vi "svl_Log View for Energy Level (single value).vi"(6 "include weighting if dB On FALSE":bool=TRUE, 7 "channel info":T1={"sensor sensitivity"=1000.0, "engineering units"=0, "dB reference"=0.0, "custom label"="EU", "weighting filter"=0, "pregain"=0.0} {"pregain" format="%.2f"; "weighting filter" items=["Linear", "A-weighting", "B-weighting", "C-weighting", "ITU-R 468-4", "Dolby", "CCITT", "C-message", "Wb", "Wc", "Wd", "We", "Wf", "Wh", "Wj", "Wk", "Wm", "AES17 20 kHz lowpass", "AES17 40 kHz lowpass", "AES17 20 kHz highpass", "AES17 40 kHz highpass"]; "dB reference" format="%^.1e"; "engineering units" items=["custom..."=0, "V"=1, "A"=21, "C"=30, "pC"=31, "s"=32, "-"=29, "Pa"=2, "N"=20, "g"=3, "m/s^2"=4, "m/s"=5, "m"=6, "mm/s"=12, "mm"=13, "micron/s"=14, "micron"=15, "in/s^2"=7, "in/s"=8, "in"=9, "mil/s"=10, "mil"=11, "rad/s^2"=16, "rad/s"=17, "rad"=18, "deg/s^2"=26, "deg/s"=27, "deg"=28, "RPM"=22, "cycle/s^2"=23, "Hz"=24, "cycle"=25, "strain"=19]; "sensor sensitivity" format="%#_5f"}, 8 "error in (no error)":errorcluster, 9 "view mode":enum16{"Power", "Amplitude"}(ring), 10 "dB On (T)":bool=TRUE, 11 "energy level [EU^2 rms]":dbl format="%.2f") -> (0 "error out":errorcluster, 2 "unit label":string, 3 "energy level [EU^2 rms]":dbl format="%.2f")   [LabVIEW 2017]
uses:
  <vilib>/addons/_NISVFA/_Shared subVIs/Controls/svc_Channel Info.ctl
  <vilib>/addons/_NISVFA/_Shared subVIs/Controls/svc_Engineering Units Text Ring.ctl
  <vilib>/addons/_NISVFA/_Shared subVIs/Controls/svc_Weighting Filter Text Ring.ctl
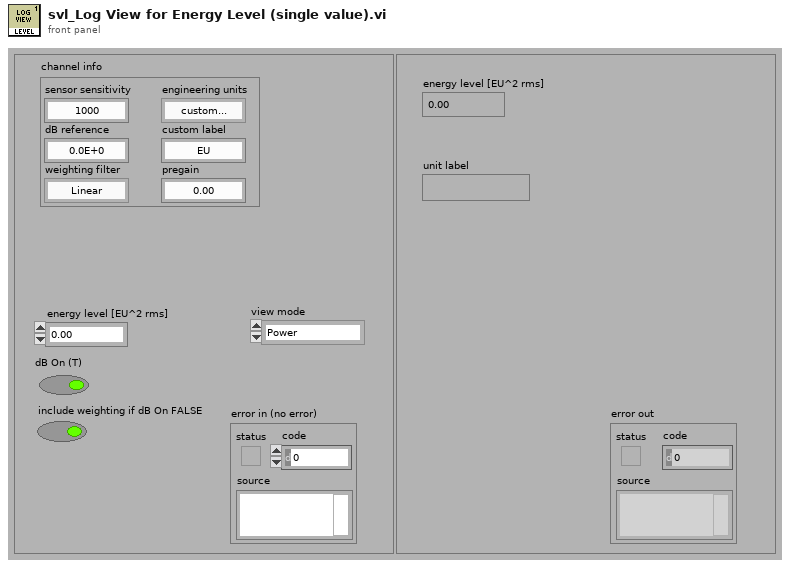
[diagram p1: front panel]
types:
  T1 = typedef "svc_Channel Info.ctl" = cluster{"sensor sensitivity":dbl, "engineering units":T2, "dB reference":dbl, "custom label":string, "weighting filter":T3, "pregain":dbl}
  T2 = typedef "svc_Engineering Units Text Ring.ctl" = u16
  T3 = typedef "svc_Weighting Filter Text Ring.ctl" = u16
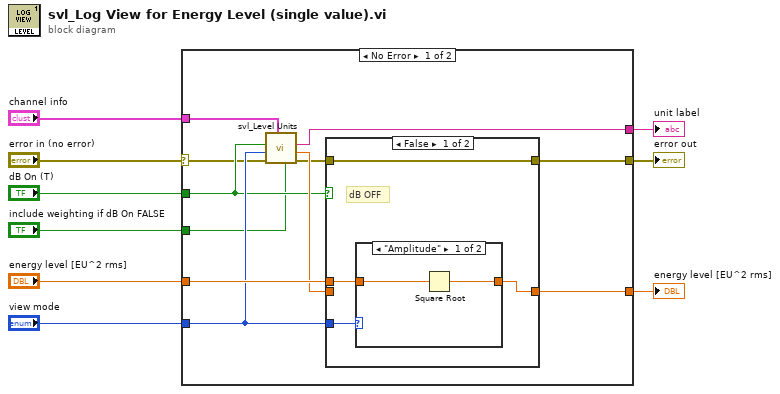
[diagram p0: block diagram]
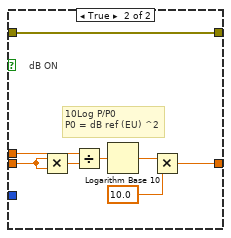
[diagram p3: hidden frame]
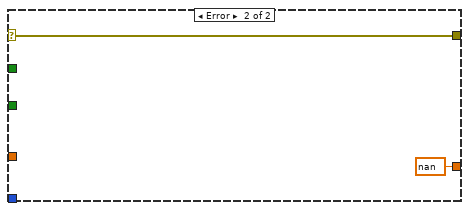
[diagram p4: hidden frame]
diagram:
  n1 = case shown="No Error" "error in (no error)" {
    selector: "error in (no error)" -> [w10 w37]
    tunnel: "energy level [EU^2 rms]" -> [w20 _]
    tunnel: [w19 nan ("energy level [EU^2 rms]")] -> w8
    tunnel: [w16 w37] -> w7
    tunnel: "view mode" -> [w15 _]
    tunnel: "dB On (T)" -> [w14 _]
    tunnel: "include weighting if dB On FALSE" -> [w13 _]
    tunnel: "channel info" -> [w12 _]
    tunnel: [w11 _] -> w2
    frame No Error {
      n2 = call <vilib>:"svl_Level Units.vi"("include weighting if dB On FALSE"=w13, "channel info"=w12, "error in (no error)"=w10, "view mode"=w15, "dB On (T)"=w14) -> ("error out"=w17:errorcluster, "dB reference [EU]"=w18:dbl, "unit label"=w11:string)  [unwired: 4 in]
      n3 = case shown="False" w14 {
        tunnel: [w24 w35] -> w19
        tunnel: w20 -> [w22 w34]
        tunnel: w15 -> [w23 _]
        tunnel: w18 -> [_ w29]
        tunnel: w17 -> [w21 w28]
        tunnel: [w21 w28] -> w16
        frame False {
          # "dB OFF"
          n4 = case shown="\"Amplitude\"" w23 {
            tunnel: [w26 w27] -> w24
            tunnel: w22 -> [w25 w27]
            frame "Amplitude" {
              n5 = Square Root(x=w25) -> (sqrt(x)=w26:dbl)
            }
            frame "Power", Default {
            }
          }
        }
        frame True {
          # "10Log P/P0\nP0 = dB ref (EU) ^2"
          # "dB ON"
          n6 = Multiply(x=w29, y=w29) -> (x*y=w30:dbl)
          n7 = Divide(x=w34, y=w30) -> (x/y=w31:dbl)
          n8 = Logarithm Base 10(1:w31) -> (0:w32:dbl)
          n9 = Multiply(x=w32, y=10.0) -> (x*y=w35:dbl)
        }
      }
    }
    frame Error {
    }
  }
  "unit label" <- w2
  "energy level [EU^2 rms]" <- w8
  "error out" <- w7
